vi "N_Trig.vi"(11 "In":bool) -> (3 "Q":bool)   [LabVIEW 2020]
panel:
  out "Memory bit":bool
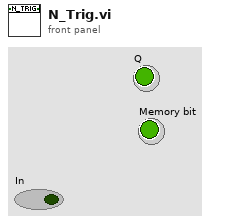
[diagram p1: front panel]
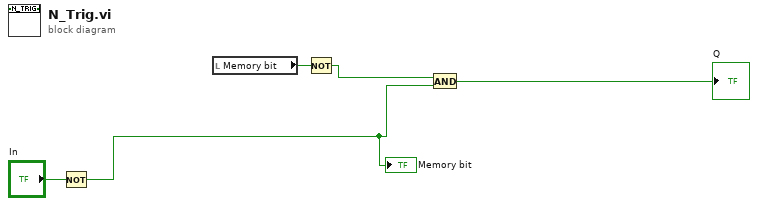
[diagram p0: block diagram]
diagram:
  n1 = Not(x="In") -> (.not. x?=w2:bool)
  "Memory bit" <- w2
  n2 = local read "Memory bit"() -> (w1:bool)
  n3 = Not(x=w1) -> (.not. x?=w5:bool)
  n4 = And(x=w5, y=w2) -> (x .and. y?=→"Q":bool)
